vi "Marker Types.vi"() -> (1 "Cancel":bool=TRUE, 3 "Type":T1(ring)=enum."vert")   [LabVIEW 2015]
uses:
  <vilib>/Utility/miscctls.llb/LVRectTypeDef.ctl
  <vilib>/Utility/inputDevices.llb/mouseAcquire.vi
panel:
  in  "Box Range":bool
  in  "Horizontal Range":bool
  in  "Verticle Range":bool
  in  "Verticle Line":bool
  in  "Horizontal Line":bool
  in  "Point":bool
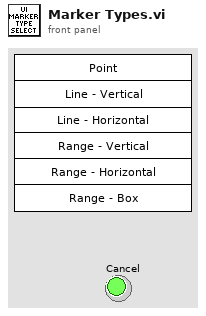
[diagram p1: front panel]
types:
  T1 = enum16{"point", "horiz", "vert", "vert range", "horiz range", "box"}
  T2 = typedef "LVRectTypeDef.ctl" = cluster{"Left":i16, "Top":i16, "Right":i16, "Bottom":i16}
  T3 = cluster{"Horizontal":i32, "Vertical":i32, "Scrolling":i32}
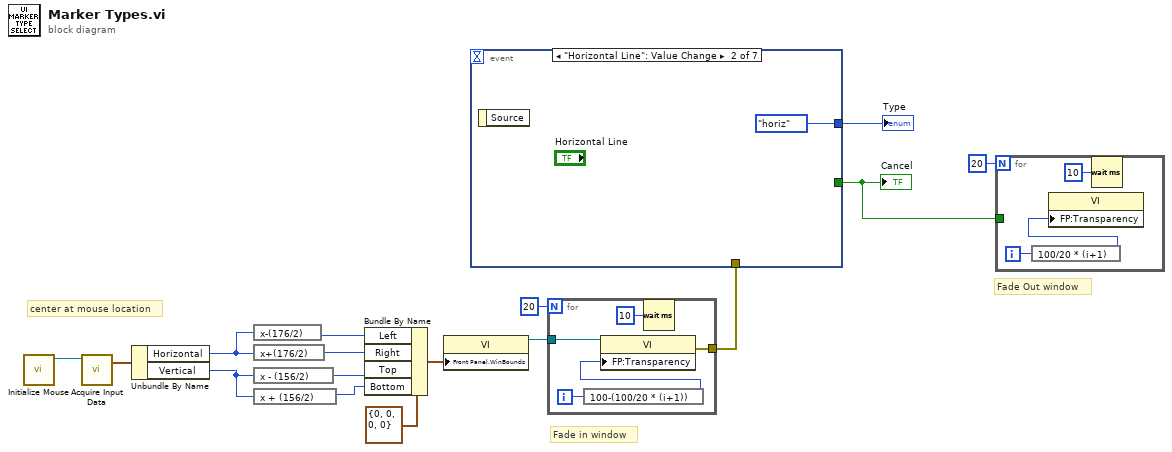
[diagram p0: block diagram]
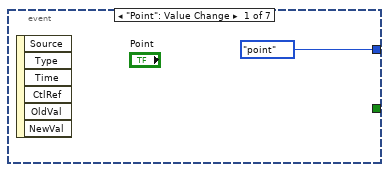
[diagram p2: hidden frame]
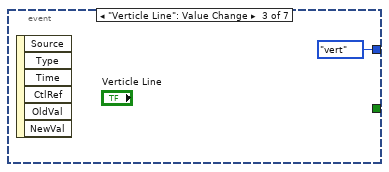
[diagram p3: hidden frame]
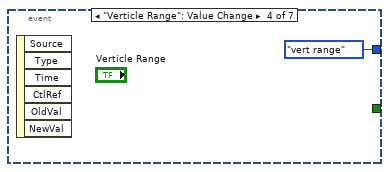
[diagram p4: hidden frame]
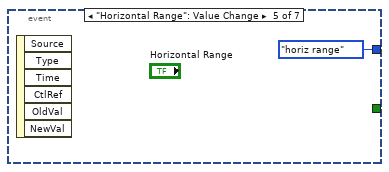
[diagram p5: hidden frame]
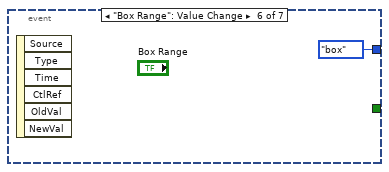
[diagram p6: hidden frame]
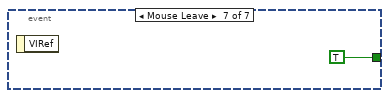
[diagram p7: hidden frame]
diagram:
  # "Fade Out window"
  # "Fade in window"
  # "center at mouse location"
  n1 = call <vilib>:"Initialize Mouse.vi"() -> ("device ID"=w15:refnum<k1>)  [unwired: 10 in, 1 out]
  n2 = call-poly <vilib>:"Acquire Input Data.vi"("device ID"=w15) -> ("axis info"=w14:T3)  [unwired: 15 in, 3 out]
  n3 = Unbundle By Name(w14) -> ("Horizontal"=w7:i32, "Vertical"=w8:i32)
  n4 = expression code="x-(176/2)"(w7) -> (w11:i32)
  n5 = expression code="x+(176/2)"(w7) -> (w12:i32)
  n6 = expression code="x - (156/2)"(w8) -> (w10:i32)
  n7 = expression code="x + (156/2)"(w8) -> (w9:i32)
  n8 = Bundle By Name(cluster=T2 {"Left"=0, "Top"=0, "Right"=0, "Bottom"=0} ("Front Panel Window:Window Bounds"), "Left"=w11, "Right"=w12, "Top"=w10, "Bottom"=w9) -> (w6:T2)
  n9 = property class="VI"("Front Panel.WinBounds"=w6) -> (reference out=w5:refnum<vi>)  [unwired: 2 in, 1 out]
  n10 = for {
    N: 20 -> [_]
    tunnel: w5 -> [w21]
    tunnel: [w17] -> w3
    i -> [w20]
    n11 = expression code="100-(100/20 * (i+1))"(w20) -> (w19:i32)
    n12 = property class="VI"(reference=w21, "FP:Transparency"=w19) -> (error out=w17:errorcluster)  [unwired: 1 in, 1 out]
    n13 = Wait (ms)(milliseconds to wait=u32 10) -> ()  [unwired: 1 out]
  }
  n14 = event shown="[1] \"Horizontal Line\": Value Change" {
    selector: _ -> [_ _ _ _ _ _ _]
    dyn-events: _ -> [_ _ _ _ _ _ _]
    timeout: _ -> [_ _ _ _ _ _ _]
    tunnel: [T1."point" ("Type") T1."horiz" ("Type") T1."vert" ("Type") T1."vert range" ("Type") T1."horiz range" ("Type") T1."box" ("Type") _] -> w16
    tunnel: [_ _ _ _ _ _ TRUE] -> w1
    tunnel: w3 -> [_ _ _ _ _ _ _]
    event "Point": Value Change {
      n15 = event-data() -> ()  [unwired: 1 in, 6 out]
    }
    event "Horizontal Line": Value Change {
      n16 = event-data() -> ()  [unwired: 1 in, 1 out]
    }
    event "Verticle Line": Value Change {
      n17 = event-data() -> ()  [unwired: 1 in, 6 out]
    }
    event "Verticle Range": Value Change {
      n18 = event-data() -> ()  [unwired: 1 in, 6 out]
    }
    event "Horizontal Range": Value Change {
      n19 = event-data() -> ()  [unwired: 1 in, 6 out]
    }
    event "Box Range": Value Change {
      n20 = event-data() -> ()  [unwired: 1 in, 6 out]
    }
    event Mouse Leave {
      n21 = event-data() -> ()  [unwired: 1 in, 1 out]
    }
  }
  "Type" <- w16
  "Cancel" <- w1
  n22 = for {
    N: 20 -> [_]
    tunnel: w1 -> [_]
    i -> [w31]
    n23 = expression code="100/20 * (i+1)"(w31) -> (w30:i32)
    n24 = property class="VI"("FP:Transparency"=w30) -> ()  [unwired: 2 in, 2 out]
    n25 = Wait (ms)(milliseconds to wait=u32 10) -> ()  [unwired: 1 out]
  }
